vi "RegisterProcess.vi"(8 "error in (no error)":errorcluster, 9 "Process Name (Optional)":string, 10 "Process VI (Static VI Ref)":refnum<vi>, 11 "pSubSystem in":refnum<class "JKI SMO.lvclass">) -> (0 "error out":errorcluster, 3 "pSubSystem dup":refnum<class "JKI SMO.lvclass">)   [LabVIEW 2013, in "JKI SMO.lvclass"]
doc: "---------------------------------------------------------------\nCopyright © 2014 JKI All rights reserved.\nAuthor: Philippe Guerit <philippe.guerit@jki.net>\nThis library is provided \"AS IS\" , WITHOUT WARRANTIES OR \nCONDITIONS OF ANY KIND, either express or implied.\nJKI. -- jki.net"
uses:
  JKI SMO.lvclass
  JKI SMO.lvclass/JKI SMO.ctl
panel:
  # "Copyright © 2014 JKI All rights reserved.\n\nAuthor: Philippe Guerit <philippe.guerit@jki.net>\n\nThis library is provided \"AS IS\" , WITHOUT WARRANTIES OR \nCONDITIONS OF ANY KIND, either express or implied.\n\nJKI. -- jki.net"
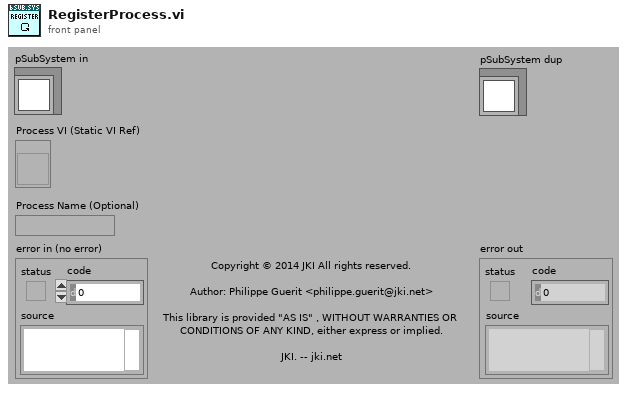
[diagram p1: front panel]
types:
  T1 = typedef "BaseSubSystem.lvclass/PrivateData--Cluster.ctl" = cluster{"Processes Clone VI Ref [ ]":refnum<vi>[], "Processes Clone Name [ ]":string[], "Process Sync RendezVous":T2, "Protected Events":T3, "Registered Process [ ]":T4[]}
  T2 = typedef "Rendezvous RefNum" = refnum<k1>
  T3 = typedef "BaseSubSystem.lvclass/ProtectedEvents--Cluster.ctl" = cluster{"StopProcesses":refnum<user-event>, "AbortProcesses":refnum<user-event>}
  T4 = typedef "BaseSubSystem.lvclass/RegisteredProcessData--Cluster.ctl" = cluster{"Name":string, "Static VI Ref":refnum<vi>}
  T5 = cluster{"Process Name (Optional)":string, "Process VI (Static VI Ref)":refnum<vi>}
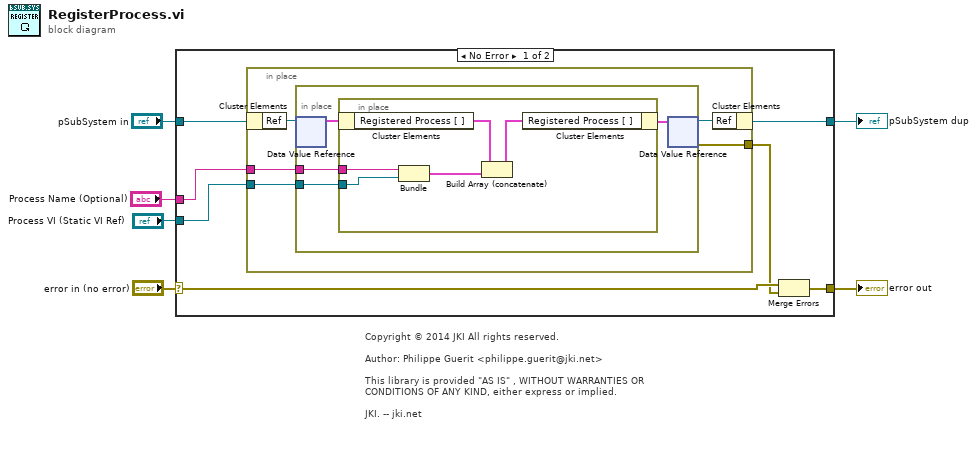
[diagram p0: block diagram]
diagram:
  # "Copyright © 2014 JKI All rights reserved.\n\nAuthor: Philippe Guerit <philippe.guerit@jki.net>\n\nThis library is provided \"AS IS\" , WITHOUT WARRANTIES OR \nCONDITIONS OF ANY KIND, either express or implied.\n\nJKI. -- jki.net"
  n1 = case shown="No Error" "error in (no error)" {
    selector: "error in (no error)" -> [w9 w29]
    tunnel: "Process VI (Static VI Ref)" -> [w11 _]
    tunnel: [w7 w29] -> w5
    tunnel: "Process Name (Optional)" -> [w12 _]
    tunnel: [w10 w28] -> w2
    tunnel: "pSubSystem in" -> [w13 w28]
    frame No Error {
      n2 = in-place {
        in-place-border: w12 -> [w17]
        in-place-border: w11 -> [w16]
        in-place-border: [w14] -> w8
        n3 = in-place-cluster #1(w13) -> ("Ref"=w18:refnum<data-value>)
        n4 = in-place {
          in-place-border: w17 -> [w21]
          in-place-border: w16 -> [w20]
          n5 = in-place-dvr #2(w18) -> (w22:T1)  [unwired: 1 out]
          n6 = in-place {
            in-place-border: w21 -> [w25]
            in-place-border: w20 -> [w24]
            n7 = in-place-cluster #3(w22) -> ("Registered Process [ ]"=w27:T4[])
            n8 = Bundle("Process Name (Optional)"=w25, "Process VI (Static VI Ref)"=w24) -> (w23:T5)  [unwired: 1 in]
            n9 = Build Array (concatenate)(w27, w23) -> (w26:T4[])
            n10 = in-place-cluster #3("Registered Process [ ]"=w26) -> (w19:T1)
          }
          n11 = in-place-dvr #2(w19) -> (w15:refnum<data-value>, w14:errorcluster)
        }
        n12 = in-place-cluster #1("Ref"=w15) -> (w10:refnum<class "JKI SMO.lvclass">)
      }
      n13 = Merge Errors(w9, w8) -> (w7:errorcluster)
    }
    frame Error {
    }
  }
  "error out" <- w5
  "pSubSystem dup" <- w2
